vi "Select Instrument Class.vi"(8 "error in":errorcluster, 9 "Instrument Class":string="Hardware Abstraction.lvlibp:NI Switch.lvclass", 10 "Instrument":T1, 11 "HAL Base Path":path=path "C:/Workspace/PPLs/Hardware Abstraction.lvlibp") -> (0 "error out":errorcluster, 3 "Class Ref":refnum<class>)   [LabVIEW 2019, in "Code Modules.lvlib"]
uses:
  PPLs/Hardware Abstraction.lvlibp/Harware Abstraction/DIO/DIO.lvclass
  C:/Workspace/PPLs/Hardware Abstraction.lvlibp/Harware Abstraction/Instrument/Instrument.lvclass
  PPLs/Hardware Abstraction.lvlibp/Harware Abstraction/Switch/Switch.lvclass
  PPLs/Hardware Abstraction.lvlibp/Harware Abstraction/MultiIO/MIO.lvclass
  Code Modules.lvlib
  <vilib>/Utility/LVLibp/NI_PackedLibraryUtility.lvlib
  PPLs/Hardware Abstraction.lvlibp/Harware Abstraction/Analog In/Analog In.lvclass
  PPLs/Hardware Abstraction.lvlibp/Harware Abstraction/Instrument/Instrument.lvclass
  Instrument -Enum.ctl
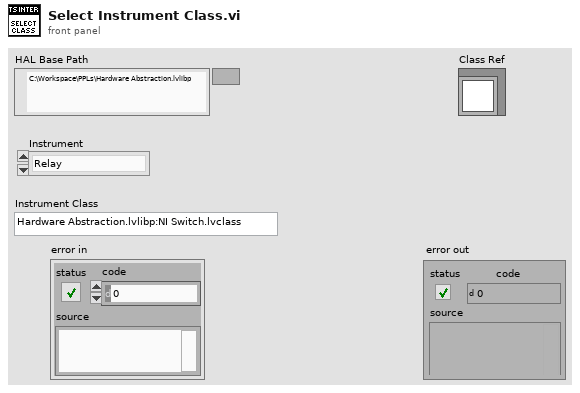
[diagram p1: front panel]
types:
  T1 = typedef "Code Modules.lvlib/Instrument -Enum.ctl" = enum16{"Relay", "MUX", "DMM", "Analog In"}
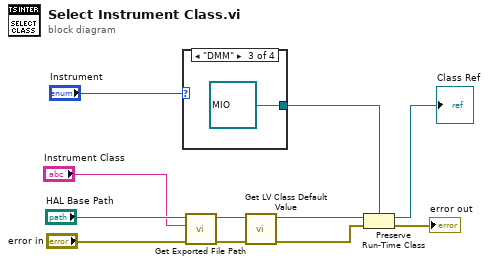
[diagram p0: block diagram]
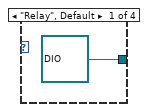
[diagram p2: hidden frame]
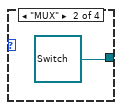
[diagram p3: hidden frame]
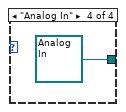
[diagram p4: hidden frame]
diagram:
  n1 = case shown="\"DMM\"" "Instrument" {
    tunnel: [refnum<class "DIO.lvclass"> refnum ("Hardware Abstraction.lvlibp:DIO.lvclass") refnum<class "Switch.lvclass"> refnum ("Hardware Abstraction.lvlibp:Switch.lvclass") refnum<class "MIO.lvclass"> refnum ("Hardware Abstraction.lvlibp:MIO.lvclass") refnum<class "Analog In.lvclass"> refnum ("Hardware Abstraction.lvlibp:Analog In.lvclass")] -> w7
    frame "Relay", Default {
    }
    frame "MUX" {
    }
    frame "DMM" {
    }
    frame "Analog In" {
    }
  }
  n2 = call <vilib>:"Get Exported File Path.vi"("error in (no error)"="error in", "qualified name"="Instrument Class", "packed library path"="HAL Base Path") -> ("error out"=w5:errorcluster, "path"=w4:path)  [unwired: 7 in]
  n3 = call <vilib>:"Get LV Class Default Value.vi"("error in (no error)"=w5, "class path"=w4) -> ("error out"=w10:errorcluster, "object"=w8:refnum<class>)  [unwired: 8 in]
  n4 = Preserve Run-Time Class(object in=w8, error in=w10, 2:w7) -> (object out=→"Class Ref":refnum<class "Instrument.lvclass">, error out=→"error out":errorcluster)
